vi "Get Class Default Object.vi"(8 "Error In":errorcluster, 11 "Class":string) -> (0 "Error Out":errorcluster, 3 "Class Default Object":refnum<class>)   [LabVIEW 2016, in "CS++Utilities.lvlib"]
doc: "Get class default object.\n\nThis VI checks if the specified class file exists and creates a default object from this path if true.\nOtherwise it assumes that the class is already loaded into memory and creates a default object specified by [Libname.lvlib:]Classname.lvclass."
uses:
  CS++Utilities.lvlib
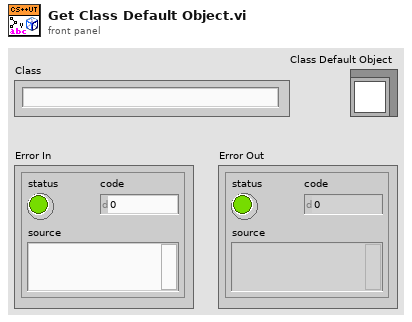
[diagram p1: front panel]
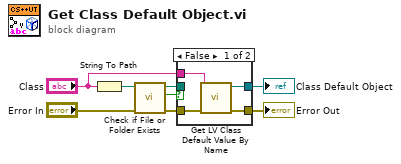
[diagram p0: block diagram]
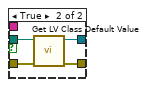
[diagram p2: hidden frame]
diagram:
  n1 = String To Path(string="Class") -> (path=w4:path)
  n2 = call <vilib>:"Check if File or Folder Exists.vi"("error in (no error)"="Error In", "path"=w4) -> ("error out"=w6:errorcluster, "file or folder exists?"=w7:bool, "dup path"=w5:path)  [unwired: 7 in]
  n3 = case shown="False" w7 {
    tunnel: w5 -> [_ w16]
    tunnel: w6 -> [w12 w15]
    tunnel: "Class" -> [w11 _]
    tunnel: [w10 w14] -> w2
    tunnel: [w9 w13] -> w1
    frame False {
      n4 = call <vilib>:"Get LV Class Default Value By Name.vi"("error in (no error)"=w12, "class name"=w11) -> ("error out"=w10:errorcluster, "object"=w9:refnum<class>)  [unwired: 8 in]
    }
    frame True {
      n5 = call <vilib>:"Get LV Class Default Value.vi"("error in (no error)"=w15, "class path"=w16) -> ("error out"=w14:errorcluster, "object"=w13:refnum<class>)  [unwired: 8 in]
    }
  }
  "Error Out" <- w2
  "Class Default Object" <- w1
